vi "adjustAngle_00.vi"() -> ()   [LabVIEW 2011]
panel:
  in  "Move to ref angle first":bool
  in  "time done (s)":dbl
  in  "time to wait (s)":dbl
  out "Wait to set":bool
  in  "Ref Angle (deg)":dbl format="%.1f"
  out "IO error":errorcluster
  in  "stop":bool
  out "Angle Indicator (deg)":dbl caption="Angle (deg)" format="%.1f"
  in  "Angle (deg)":dbl format="%.1f"
  out "P (torr)":dbl format="%.2f"
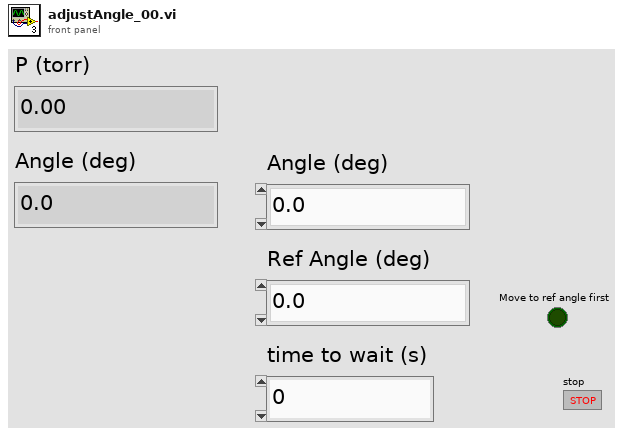
[diagram p1: front panel]
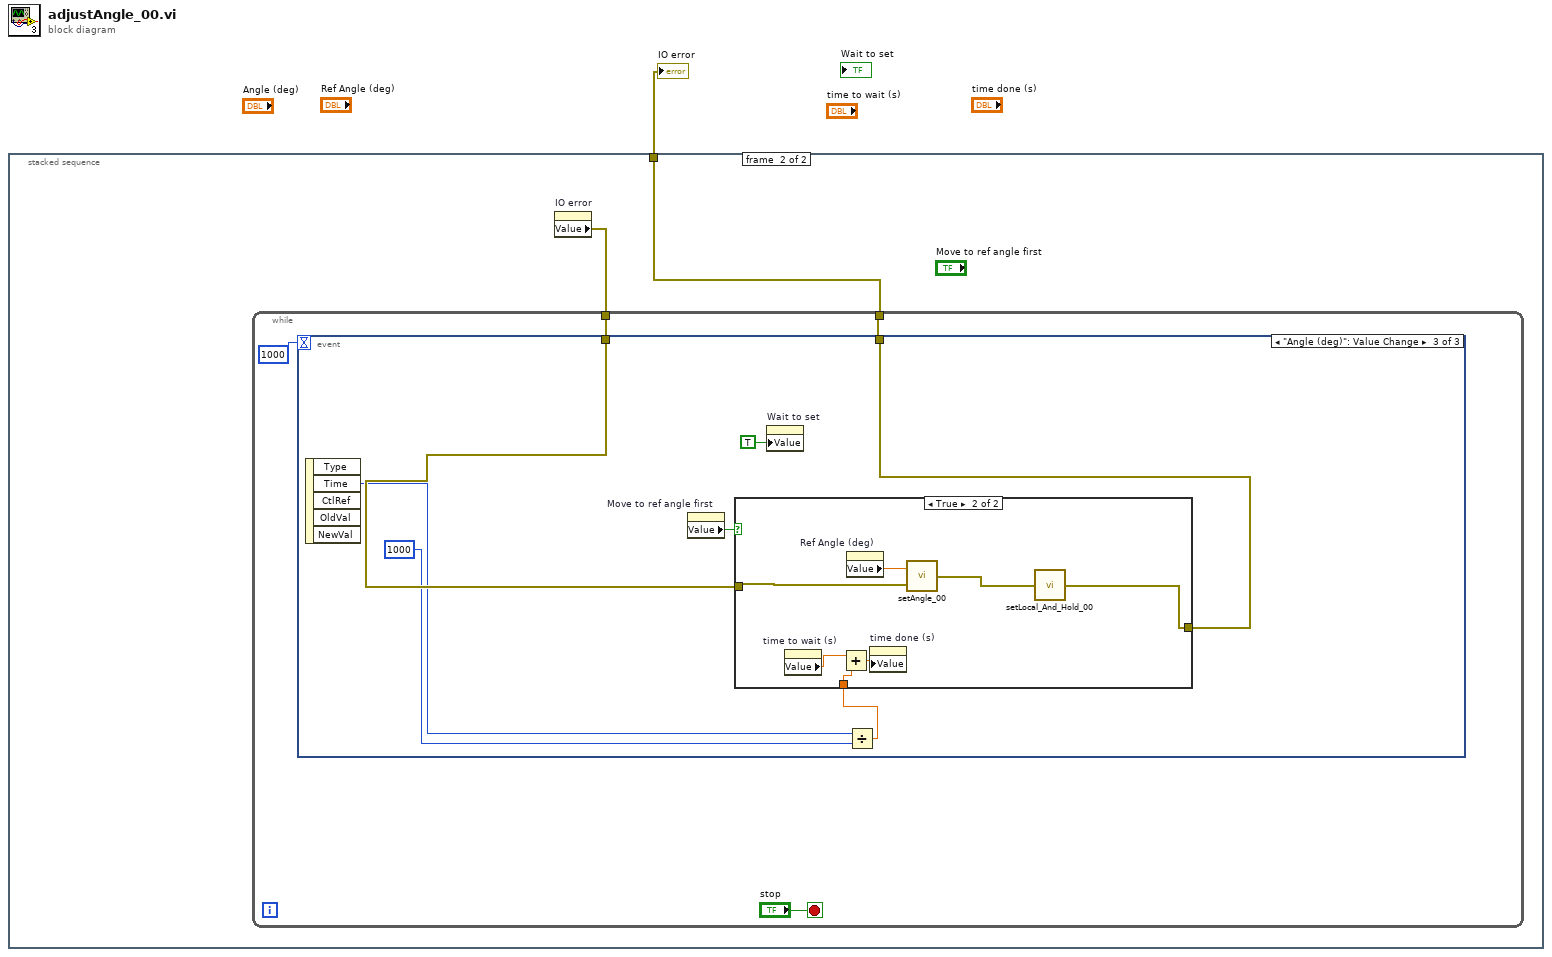
[diagram p0: block diagram]
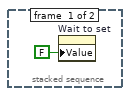
[diagram p2: hidden frame]
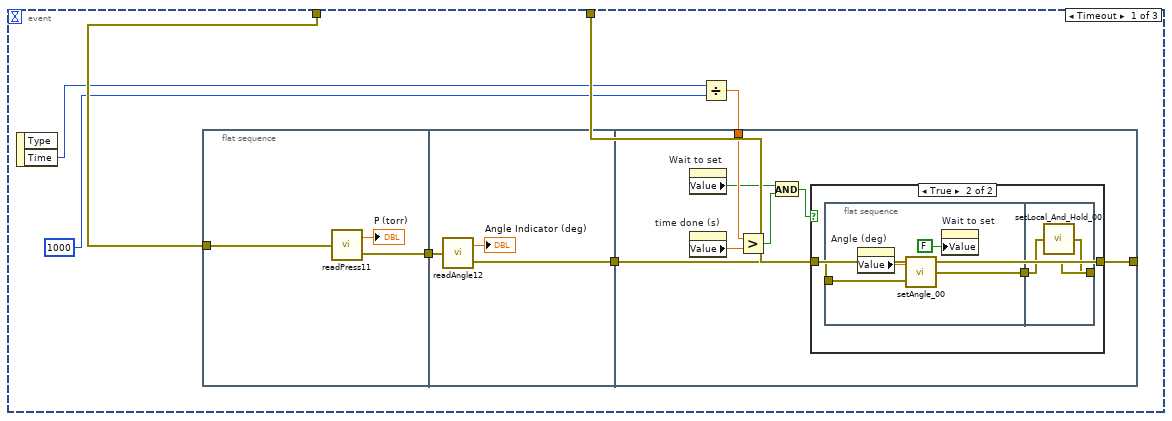
[diagram p3: hidden frame]
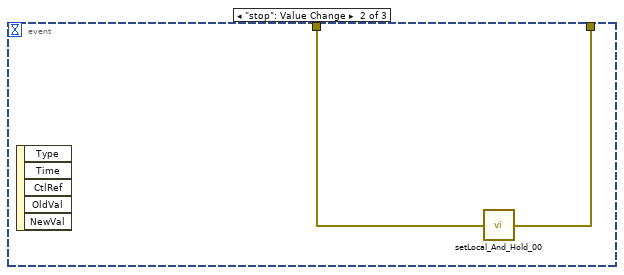
[diagram p5: hidden frame]
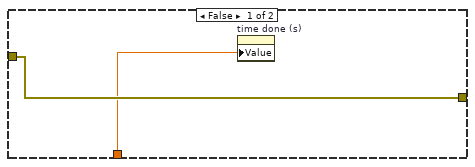
[diagram p6: hidden frame]
diagram:
  n1 = stacked-sequence {
    tunnel: [_ w3] -> w1
    frame #0 {
      n2 = property on="Wait to set" class="Bool (strict)"("Value"=FALSE ("Wait to set")) -> ()  [unwired: 2 in, 2 out]
    }
    frame #1 {
      n3 = property on="IO error" class="Clust (strict)"() -> ("Value"=w4:errorcluster)  [unwired: 2 in, 2 out]
      n4 = while {
        tunnel: w4 -> [w7]
        tunnel: [w6] -> w3
        stop <- "stop" stop-if-true
        n5 = event shown="[2] \"Angle (deg)\": Value Change" {
          selector: _ -> [_ _ _]
          dyn-events: _ -> [_ _ _]
          timeout: 1000 -> [_ _ _]
          tunnel: w7 -> [w15 w40 w46]
          tunnel: [w12 w39 w47] -> w6
          event Timeout {
            n6 = event-data() -> ("Time"=w11:u32)  [unwired: 1 in, 1 out]
            n7 = flat-sequence {
              tunnel: w15 -> [w18]
              tunnel: [w17] -> w14
              tunnel: w14 -> [w21]
              tunnel: [w19] -> w13
              tunnel: w9 -> [w28]
              tunnel: w13 -> [w24]
              tunnel: [w23] -> w12
              frame #0 {
                n8 = call "readPress11.vi"("error in"=w18) -> ("P"=→"P (torr)":dbl, "error out"=w17:errorcluster)
              }
              frame #1 {
                n9 = call "readAngle12.vi"("error in"=w21) -> ("angle"=→"Angle Indicator (deg)":dbl, "error out"=w19:errorcluster)
              }
              frame #2 {
                n10 = property on="Wait to set" class="Bool (strict)"() -> ("Value"=w22:bool)  [unwired: 2 in, 2 out]
                n11 = property on="time done (s)" class="DigNum (strict)"() -> ("Value"=w27:dbl)  [unwired: 2 in, 2 out]
                n12 = Greater?(x=w28, y=w27) -> (0:w26:bool)
                n13 = And(x=w22, y=w26) -> (x .and. y?=w25:bool)
                n14 = case shown="True" w25 {
                  tunnel: w24 -> [w29 w32]
                  tunnel: [w29 w31] -> w23
                  frame False {
                  }
                  frame True {
                    n15 = flat-sequence {
                      tunnel: w32 -> [w35]
                      tunnel: [w34] -> w30
                      tunnel: [w37] -> w31
                      tunnel: w30 -> [w38]
                      frame #0 {
                        n16 = property on="Angle (deg)" class="DigNum (strict)"() -> ("Value"=w36:dbl)  [unwired: 2 in, 2 out]
                        n17 = call "setAngle_00.vi"("error in (no error)"=w35, "Angle (deg)"=w36) -> ("error out"=w34:errorcluster)
                        n18 = property on="Wait to set" class="Bool (strict)"("Value"=FALSE ("Wait to set")) -> ()  [unwired: 2 in, 2 out]
                      }
                      frame #1 {
                        n19 = call "setLocal_And_Hold_00.vi"("error in (no error)"=w38) -> ("error out"=w37:errorcluster)
                      }
                    }
                  }
                }
              }
            }
            n20 = Divide(x=w11, y=u32 1000) -> (x/y=w9:dbl)
          }
          event "stop": Value Change {
            n21 = event-data() -> ()  [unwired: 1 in, 5 out]
            n22 = call "setLocal_And_Hold_00.vi"("error in (no error)"=w40) -> ("error out"=w39:errorcluster)
          }
          event "Angle (deg)": Value Change {
            n23 = event-data() -> ("Time"=w45:u32)  [unwired: 1 in, 4 out]
            n24 = property on="Move to ref angle first" class="Bool (strict)"() -> ("Value"=w42:bool)  [unwired: 2 in, 2 out]
            n25 = property on="Wait to set" class="Bool (strict)"("Value"=TRUE ("Wait to set")) -> ()  [unwired: 2 in, 2 out]
            n26 = Divide(x=w45, y=u32 1000) -> (x/y=w43:dbl)
            n27 = case shown="True" w42 {
              tunnel: w46 -> [w49 w55]
              tunnel: [w49 w50] -> w47
              tunnel: w43 -> [w48 w52]
              frame False {
                n28 = property on="time done (s)" class="DigNum (strict)"("Value"=w48) -> ()  [unwired: 2 in, 2 out]
              }
              frame True {
                n29 = property on="time to wait (s)" class="DigNum (strict)"() -> ("Value"=w53:dbl)  [unwired: 2 in, 2 out]
                n30 = Add(x=w53, y=w52) -> (x+y=w54:dbl)
                n31 = property on="Ref Angle (deg)" class="DigNum (strict)"() -> ("Value"=w56:dbl)  [unwired: 2 in, 2 out]
                n32 = property on="time done (s)" class="DigNum (strict)"("Value"=w54) -> ()  [unwired: 2 in, 2 out]
                n33 = call "setAngle_00.vi"("error in (no error)"=w55, "Angle (deg)"=w56) -> ("error out"=w51:errorcluster)
                n34 = call "setLocal_And_Hold_00.vi"("error in (no error)"=w51) -> ("error out"=w50:errorcluster)
              }
            }
          }
        }
      }
    }
  }
  "IO error" <- w1
